vi "AnalyzePulseTrain for Closed IPG.vi"(7 "Pulse Characteristics":T2={"Pulses per Cycle"=4, "Load Resistance (Ohms)"=nan, "Krec Value"=2, "Recovery Mode (T=Active)"=TRUE, "Target Stim Currents (Amps)"=[]}, 8 "Repetitions in the Input Waveform":i32=4, 9 "Waveform In":waveform(dbl)={"t0"=timestamp(3433165898.5470004 s since 1904-01-01), "dt"=nan, "Y"=[]}) -> (3 "Waveform Parameters":T1={"Stim Amplitude"=[], "Stim Pulse Width"=[], "Interphase Delay"=[], "Recovery Amplitude"=[], "Recovery PW"=[], "Recovery Holdoff"=[], "Frequency"=nan, "Avg CBC Width"=nan, "Avg. CBC Holdoff"=0.0, "Avg. CBC Amplitude"=nan} {"Avg. CBC Amplitude" format="%.1p"; "Frequency" format="%.1p"; "Avg CBC Width" format="%.1p"; "Avg. CBC Holdoff" format="%.1p"; "Stim Pulse Width" format="%.1p"; "Interphase Delay" format="%.1p"; "Recovery PW" format="%.1p"; "Recovery Holdoff" format="%.1p"; "Stim Amplitude" format="%.1p"; "Recovery Amplitude" format="%.1p"})   [LabVIEW 2010]
uses:
  MyCalc/Analyze Ouptut Parameters.ctl
  <vilib>/measure/mamon.llb/Trigger Detection for 1 Channel.vi
  <vilib>/measure/NI_MAPro.lvlib
  <vilib>/Analysis/NI_AALBase.lvlib
panel:
  out "Normalized Waveform":waveform(dbl)(graph)={"t0"=timestamp(3433165898.5470004 s since 1904-01-01), "dt"=1e-05, "Y"=array[4250 elements]}
  # "The input waveform should be a capture of the STIM chip output\n(before the cap) when the output is held at 1/2 HVDD by the\nLoad Resistance.  This ensures that passive recovery and CBC\npulses are captured, because they look like pulses pulled to GND."
  # "The elements in these arrays correspond to the pulses per cycle.\nThey are the averages over all the repetitions in the waveform."
  # "Enter Target Current\nfor each in array below"
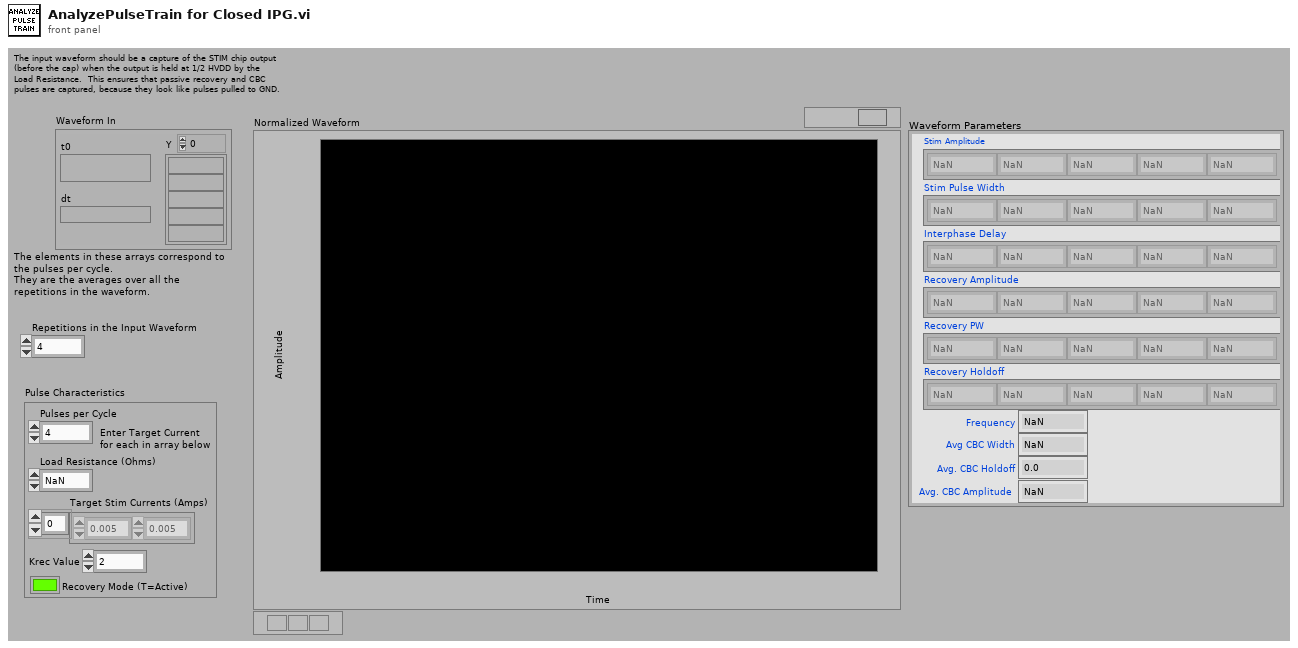
[diagram p1: front panel]
types:
  T1 = typedef "Analyze Ouptut Parameters.ctl" = cluster{"Stim Amplitude":dbl[], "Stim Pulse Width":dbl[], "Interphase Delay":dbl[], "Recovery Amplitude":dbl[], "Recovery PW":dbl[], "Recovery Holdoff":dbl[], "Frequency":dbl, "Avg CBC Width":dbl, "Avg. CBC Holdoff":dbl, "Avg. CBC Amplitude":dbl}
  T2 = cluster{"Pulses per Cycle":i32, "Load Resistance (Ohms)":dbl, "Krec Value":i32, "Recovery Mode (T=Active)":bool, "Target Stim Currents (Amps)":dbl[]}
  T3 = cluster{"trigger slope":u16, "Trigger Level":dbl}[]
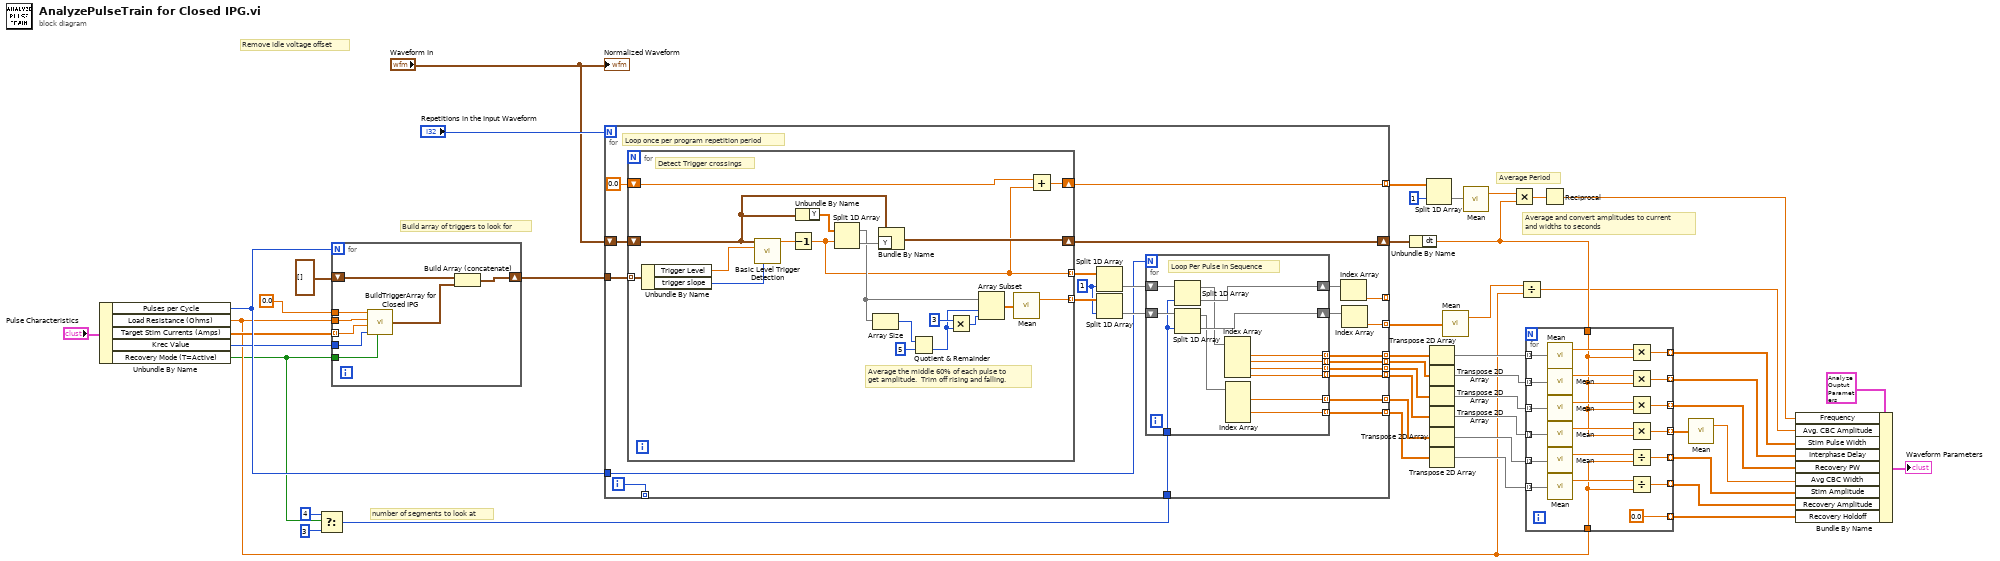
[diagram p0: block diagram]
diagram:
  # "number of segments to look at"
  # "Average Period"
  # "Average and convert amplitudes to current\nand widths to seconds"
  # "Build array of triggers to look for"
  # "Remove idle voltage offset"
  n1 = Unbundle By Name("Pulse Characteristics") -> ("Pulses per Cycle"=w32:i32, "Load Resistance (Ohms)"=w26:dbl, "Target Stim Currents (Amps)"=w31:dbl[], "Krec Value"=w30:i32, "Recovery Mode (T=Active)"=w11:bool)
  n2 = Select(t=4, s=w11, f=3 ("index")) -> (s? t:f=w9:i32)
  n3 = for {
    N: w32 -> [_]
    shift-right: [w55] -> w13
    shift-left: T3 [] -> [w54]
    tunnel: 0.0 ("mean") -> [w53]
    tunnel: w11 -> [w52]
    tunnel: w26 -> [w51]
    tunnel: w31 -> [w50] mode=indexing
    tunnel: w30 -> [w49]
    n4 = call "BuildTriggerArray for Closed IPG.vi"("CBC Trigger Level"=w53, "Load Resistance (Ohms)"=w51, "Target Stim Current (Amps)"=w50, "Krec Value"=w49, "Recovery Mode (T=Active)"=w52) -> ("Pulse Triggers"=w48:T3)
    n5 = Build Array (concatenate)(w54, w48) -> (w55:T3)
  }
  n6 = for {
    N: "Repetitions in the Input Waveform" -> [_]
    tunnel: w13 -> [w78]
    shift-right: [w74] -> w28
    shift-left: "Waveform In" -> [w77]
    tunnel: w32 -> [w71]
    tunnel: [w68] -> _ mode=indexing
    tunnel: [w67] -> w45 mode=indexing
    tunnel: [w66] -> w44 mode=indexing
    tunnel: [w65] -> w43 mode=indexing
    tunnel: [w64] -> w42 mode=indexing
    tunnel: [w63] -> w41 mode=indexing
    tunnel: [w62] -> w40 mode=indexing
    tunnel: [w61] -> w39 mode=indexing
    tunnel: [w58] -> w25 mode=indexing
    tunnel: w9 -> [w57]
    tunnel: [w56] -> _ mode=indexing
    i -> [w56]
    w75 = 1 ("index")
    # "Loop once per program repetition period"
    n7 = for {
      tunnel: w78 -> [w110] mode=indexing
      shift-right: [w96] -> w74
      shift-left: w77 -> [w105]
      tunnel: [w97] -> w76 mode=indexing
      tunnel: [w92] -> w59 mode=indexing
      shift-right: [w95] -> w58
      shift-left: 0.0 -> [w94]
      # "Detect Trigger crossings"
      # "Average the middle 60% of each pulse to\nget amplitude.  Trim off rising and falling."
      n8 = Unbundle By Name(w110) -> ("Trigger Level"=w109:dbl, "trigger slope"=w108:u16)
      n9 = call-poly <vilib>:"Basic Level Trigger Detection.vi"("signal in"=w105, "level"=w109, "trigger slope"=w108) -> ("trigger location"=w93:dbl)  [unwired: 10 in, 2 out]
      n10 = Decrement(x=w93) -> (x-1=w92:dbl)
      n11 = Unbundle By Name(w105) -> ("Y"=w107:dbl[])
      n12 = Split 1D Array(array=w107, index=w92) -> (first subarray=w99:dbl[], second subarray=w106:dbl[])
      n13 = Array Size(array=w99) -> (size(s)=w104:i32)
      n14 = Bundle By Name(cluster=w105, "Y"=w106) -> (w96:waveform(dbl))
      n15 = Quotient & Remainder(x=w104, y=5) -> (floor(x/y)=w101:i32)  [unwired: 1 out]
      n16 = Multiply(x=3, y=w101) -> (x*y=w100:i32)
      n17 = Array Subset(array=w99, index=w101, length=w100) -> (w98:dbl[])
      n18 = call <vilib>:"Mean.vi"("X"=w98) -> ("mean"=w97:dbl)  [unwired: 1 out]
      n19 = Add(x=w94, y=w92) -> (x+y=w95:dbl)
    }
    n20 = Split 1D Array(array=w59, index=w75) -> (second subarray=w73:dbl[])  [unwired: 1 out]
    n21 = Split 1D Array(array=w76, index=w75) -> (second subarray=w72:dbl[])  [unwired: 1 out]
    n22 = for {
      N: w71 -> [_]
      shift-right: [w89] -> w70
      shift-left: w73 -> [w91]
      shift-right: [w88] -> w69
      shift-left: w72 -> [w90]
      tunnel: [w85] -> w66 mode=indexing
      tunnel: [w84] -> w65 mode=indexing
      tunnel: [w83] -> w64 mode=indexing
      tunnel: [w82] -> w63 mode=indexing
      tunnel: [w81] -> w62 mode=indexing
      tunnel: [w80] -> w61 mode=indexing
      tunnel: w57 -> [w79]
      # "Loop Per Pulse in Sequence"
      n23 = Split 1D Array(array=w91, index=w79) -> (first subarray=w87:dbl[], second subarray=w89:dbl[])
      n24 = Split 1D Array(array=w90, index=w79) -> (first subarray=w86:dbl[], second subarray=w88:dbl[])
      n25 = Index Array(array=w87) -> (element #1=w85:dbl, element #2=w84:dbl, element #3=w83:dbl, element #4=w82:dbl)  [unwired: 4 in]
      n26 = Index Array(array=w86) -> (element #1=w81:dbl, element #3=w80:dbl)  [unwired: 4 in, 2 out]
    }
    n27 = Index Array(array=w70) -> (element=w68:dbl)  [unwired: 1 in]
    n28 = Index Array(array=w69) -> (element=w67:dbl)  [unwired: 1 in]
  }
  n29 = Unbundle By Name(w28) -> ("dt"=w22:dbl)
  n30 = Split 1D Array(array=w25, index=1) -> (second subarray=w24:dbl[])  [unwired: 1 out]
  n31 = Transpose 2D Array(2D array=w44) -> (transposed array=w38:dbl[][])
  n32 = Transpose 2D Array(2D array=w43) -> (transposed array=w37:dbl[][])
  n33 = Transpose 2D Array(2D array=w42) -> (transposed array=w36:dbl[][])
  n34 = Transpose 2D Array(2D array=w41) -> (transposed array=w35:dbl[][])
  n35 = Transpose 2D Array(2D array=w40) -> (transposed array=w34:dbl[][])
  n36 = Transpose 2D Array(2D array=w39) -> (transposed array=w33:dbl[][])
  n37 = call <vilib>:"Mean.vi"("X"=w45) -> ("mean"=w27:dbl)  [unwired: 1 out]
  n38 = call <vilib>:"Mean.vi"("X"=w24) -> ("mean"=w23:dbl)  [unwired: 1 out]
  n39 = Multiply(x=w23, y=w22) -> (x*y=w21:dbl)
  n40 = Divide(x=w27, y=w26) -> (x/y=w1:dbl)
  n41 = for {
    tunnel: w38 -> [w131] mode=indexing
    tunnel: w37 -> [w130] mode=indexing
    tunnel: w36 -> [w129] mode=indexing
    tunnel: w35 -> [w128] mode=indexing
    tunnel: w34 -> [w127] mode=indexing
    tunnel: w33 -> [w126] mode=indexing
    tunnel: [w125] -> w19 mode=indexing
    tunnel: [w124] -> w18 mode=indexing
    tunnel: [w123] -> w17 mode=indexing
    tunnel: [w122] -> w12 mode=indexing
    tunnel: [w121] -> w16 mode=indexing
    tunnel: [w120] -> w15 mode=indexing
    tunnel: w22 -> [w113]
    tunnel: w26 -> [w112]
    tunnel: [0.0 ("Load Resistance (Ohms)")] -> w4 mode=indexing
    n42 = call <vilib>:"Mean.vi"("X"=w131) -> ("mean"=w118:dbl)  [unwired: 1 out]
    n43 = call <vilib>:"Mean.vi"("X"=w130) -> ("mean"=w117:dbl)  [unwired: 1 out]
    n44 = call <vilib>:"Mean.vi"("X"=w129) -> ("mean"=w116:dbl)  [unwired: 1 out]
    n45 = call <vilib>:"Mean.vi"("X"=w128) -> ("mean"=w115:dbl)  [unwired: 1 out]
    n46 = call <vilib>:"Mean.vi"("X"=w127) -> ("mean"=w114:dbl)  [unwired: 1 out]
    n47 = call <vilib>:"Mean.vi"("X"=w126) -> ("mean"=w119:dbl)  [unwired: 1 out]
    n48 = Multiply(x=w118, y=w113) -> (x*y=w125:dbl)
    n49 = Multiply(x=w117, y=w113) -> (x*y=w124:dbl)
    n50 = Multiply(x=w116, y=w113) -> (x*y=w123:dbl)
    n51 = Multiply(x=w115, y=w113) -> (x*y=w122:dbl)
    n52 = Divide(x=w114, y=w112) -> (x/y=w121:dbl)
    n53 = Divide(x=w119, y=w112) -> (x/y=w120:dbl)
  }
  n54 = Reciprocal(x=w21) -> (1/x=w2:dbl)
  n55 = call <vilib>:"Mean.vi"("X"=w12) -> ("mean"=w3:dbl)  [unwired: 1 out]
  n56 = Bundle By Name(cluster=T1 {"Stim Amplitude"=[0.004971399986408228, 0.003979516450805426, 0.002975699585634962, 0.001982857180437936], "Stim Pulse Width"=[0.00050225, 0.000502, 0.00050225, 0.00050225], "Interphase Delay"=[0.000148, 0.00014774999999999999, 0.000148, 0.000148], "Recovery Amplitude"=[-0.002462903727867693, -0.002032112821995463, -0.001542882284820226, -0.001052302157905118], "Recovery PW"=[0.0006954999999999999, 0.000709, 0.00070575, 0.0006965], "Recovery Holdoff"=[0.0, 0.0, 0.0, 0.0], "Frequency"=59.9029572093209, "Avg CBC Width"=0.0009714374999999999, "Avg. CBC Holdoff"=0.0, "Avg. CBC Amplitude"=0.0} ("Waveform Parameters 2"), "Frequency"=w2, "Avg. CBC Amplitude"=w1, "Stim Pulse Width"=w19, "Interphase Delay"=w18, "Recovery PW"=w17, "Avg CBC Width"=w3, "Stim Amplitude"=w16, "Recovery Amplitude"=w15, "Recovery Holdoff"=w4) -> (→"Waveform Parameters":T1)
  "Normalized Waveform" <- "Waveform In"
